vi "ejercicio solo prueba.vi"() -> ()   [LabVIEW 2020]
panel:
  out "F  2":string
  out "F":string
  out "N":dbl
  in  "stop":bool
  in  "1":bool
  in  "TIEMPO":dbl(slide) scale=0.0..1000.0
  out "2":bool
  out "1":bool
  out "F":string
  in  "CONTRASEÑA":string
  in  "USUARIO":string
  out "P":u8(slide) scale=0.0..100.0
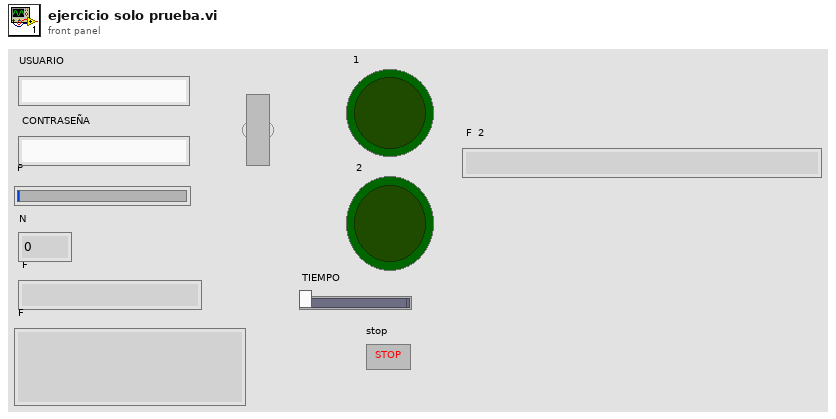
[diagram p1: front panel]
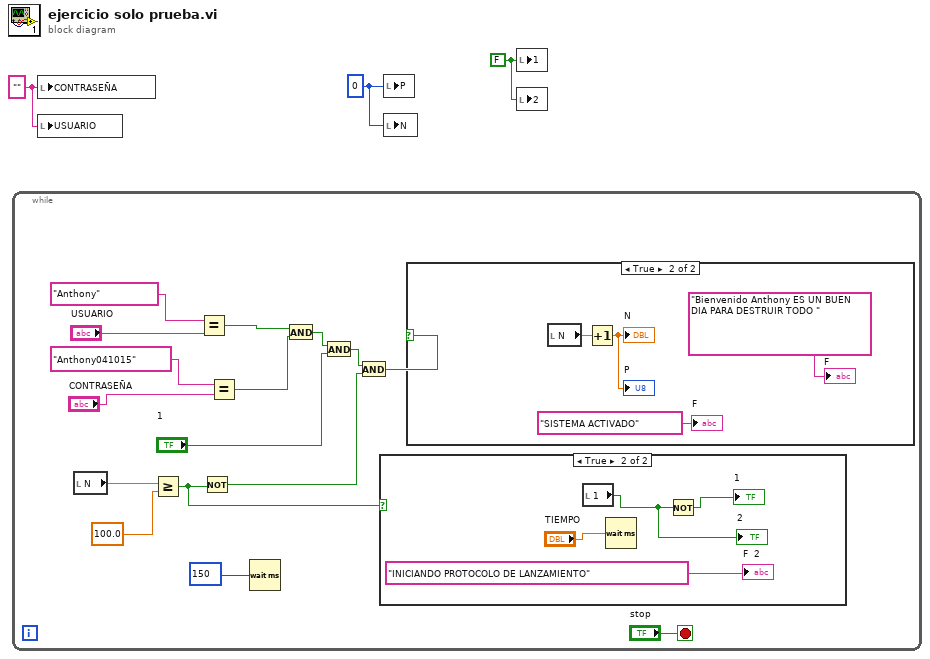
[diagram p0: block diagram]
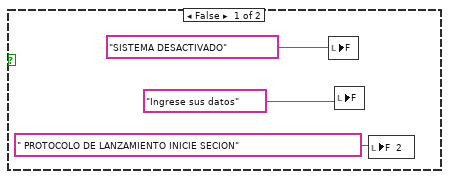
[diagram p3: hidden frame]
diagram:
  w1 = FALSE
  w2 = 0
  w3 = ""
  n1 = while {
    stop <- "stop" stop-if-true
    n2 = local read "N"() -> (w8:dbl)
    n3 = Greater Or Equal?(x=w8, y=100.0 ("x")) -> (x >= y?=w5:bool)
    n4 = Equal?(x="Anthony", y="USUARIO") -> (x = y?=w11:bool)
    n5 = Not(x=w5) -> (.not. x?=w6:bool)
    n6 = Equal?(x="Anthony041015", y="CONTRASEÑA") -> (x = y?=w12:bool)
    n7 = Wait (ms)(milliseconds to wait=u32 150 ("millisecond timer value")) -> ()  [unwired: 1 out]
    n8 = And(x=w11, y=w12) -> (x .and. y?=w14:bool)
    n9 = And(x=w14, y="1") -> (x .and. y?=w13:bool)
    n10 = And(x=w13, y=w6) -> (x .and. y?=w9:bool)
    n11 = case shown="True" w5 {
      frame False {
      }
      frame True {
        n12 = local read "1"() -> (w22:bool)
        "2" <- w22
        n13 = Wait (ms)(milliseconds to wait="TIEMPO") -> ()  [unwired: 1 out]
        n14 = Not(x=w22) -> (.not. x?=→"1":bool)
        "F  2" <- "INICIANDO PROTOCOLO DE LANZAMIENTO" ("F")
      }
    }
    n15 = case shown="True" w9 {
      frame False {
        n16 = local write "F"("SISTEMA DESACTIVADO" ("F")) -> ()
        n17 = local write "F"("Ingrese sus datos" ("F")) -> ()
        n18 = local write "F  2"(" PROTOCOLO DE LANZAMIENTO INICIE SECION" ("F")) -> ()
      }
      frame True {
        n19 = local read "N"() -> (w30:dbl)
        n20 = Increment(x=w30) -> (x+1=→"N" →"P":dbl)
        "F" <- "SISTEMA ACTIVADO" ("F")
        "F" <- "Bienvenido Anthony ES UN BUEN DIA PARA DESTRUIR TODO " ("F")
      }
    }
  }
  n21 = local write "CONTRASEÑA"(w3) -> ()
  n22 = local write "USUARIO"(w3) -> ()
  n23 = local write "P"(w2) -> ()
  n24 = local write "N"(w2) -> ()
  n25 = local write "1"(w1) -> ()
  n26 = local write "2"(w1) -> ()
